vi "vision map lines.vi"(10 "GIC Input":T2={"     Use ?\nOff       On"=[FALSE, TRUE, FALSE, TRUE], "Mode:"=FALSE, "Extra Port"="", "Hokuyo Port"="COM7", "Tx Prop  Port"="COM6", "Compass Port"="", "GPS Port"="", "Num of WPs"=0, "WP Lats and Longs"={"WP Lats"=[], "WP Longs"=[]}, "Obst Lats and Longs"={"Obst Lats"=[], "Obst Longs"=[]}, "Parameters"=[], "GPS Data"=[], "Compass"=0.0, "LMS Vector"=[], "Vision Vector"=[], "Direction Cmd"=0.0, "Speed Cmd"=0.0, "WP Vector"=[], "WP Number"=0, "Extra"=0, "SW Map"=[], "Path Cluster"={"Path x node"=[], "Path y node"=[]}, "Sim Course"=[]} {"Obst Lats and Longs"."Obst Longs" format="%#_8g"; "Obst Lats and Longs"."Obst Lats" format="%#_8g"}) -> (2 "GIC Output":T1={"     Use ?\nOff       On"=[FALSE, TRUE, FALSE, TRUE], "Mode:"=FALSE, "Extra Port"="", "Hokuyo Port"="COM7", "Tx Prop Port"="COM6", "Compass Port"="", "GPS Port"="", "Num of WPs"=0, "WP Lats and Longs"={"WP Lats"=[], "WP Longs"=[]}, "Obst Lats and Longs"={"Obst Lats"=[], "Obst Longs"=[]}, "Parameters"=[], "GPS Data"=[], "Compass"=0.0, "LMS Vector"=[], "Vision Vector"=[], "Direction Cmd"=0.0, "Speed Cmd"=0.0, "WP Vector"=[], "WP Number"=0, "Extra"=0, "SW Map"=[], "Path Cluster"={"Path x node"=[], "Path y node"=[]}, "Sim Course"=[]} {"Obst Lats and Longs"."Obst Longs" format="%#_8g"; "Obst Lats and Longs"."Obst Lats" format="%#_8g"})   [LabVIEW 2014]
panel:
  in  "y4":dbl
  in  "x4":dbl
  in  "y3":dbl
  in  "x3":dbl
  in  "y2":dbl
  in  "x2":dbl
  in  "y1":dbl
  in  "x1":dbl
  out "Local Map":picture
  out "slope":dbl
  out "yn4":dbl
  out "xn4":dbl
  out "yn3":dbl
  out "xn3":dbl
  out "yn2":dbl
  out "xn2":dbl
  out "yn1":dbl
  out "xn1":dbl
  out "th":dbl
  out "ppm":dbl
  out "yp":dbl
  out "xp":dbl
  out "SwMap out":dbl[][](array[numeric])
  # "Vision Map Lines"
  # "Input:"
  # "Output"
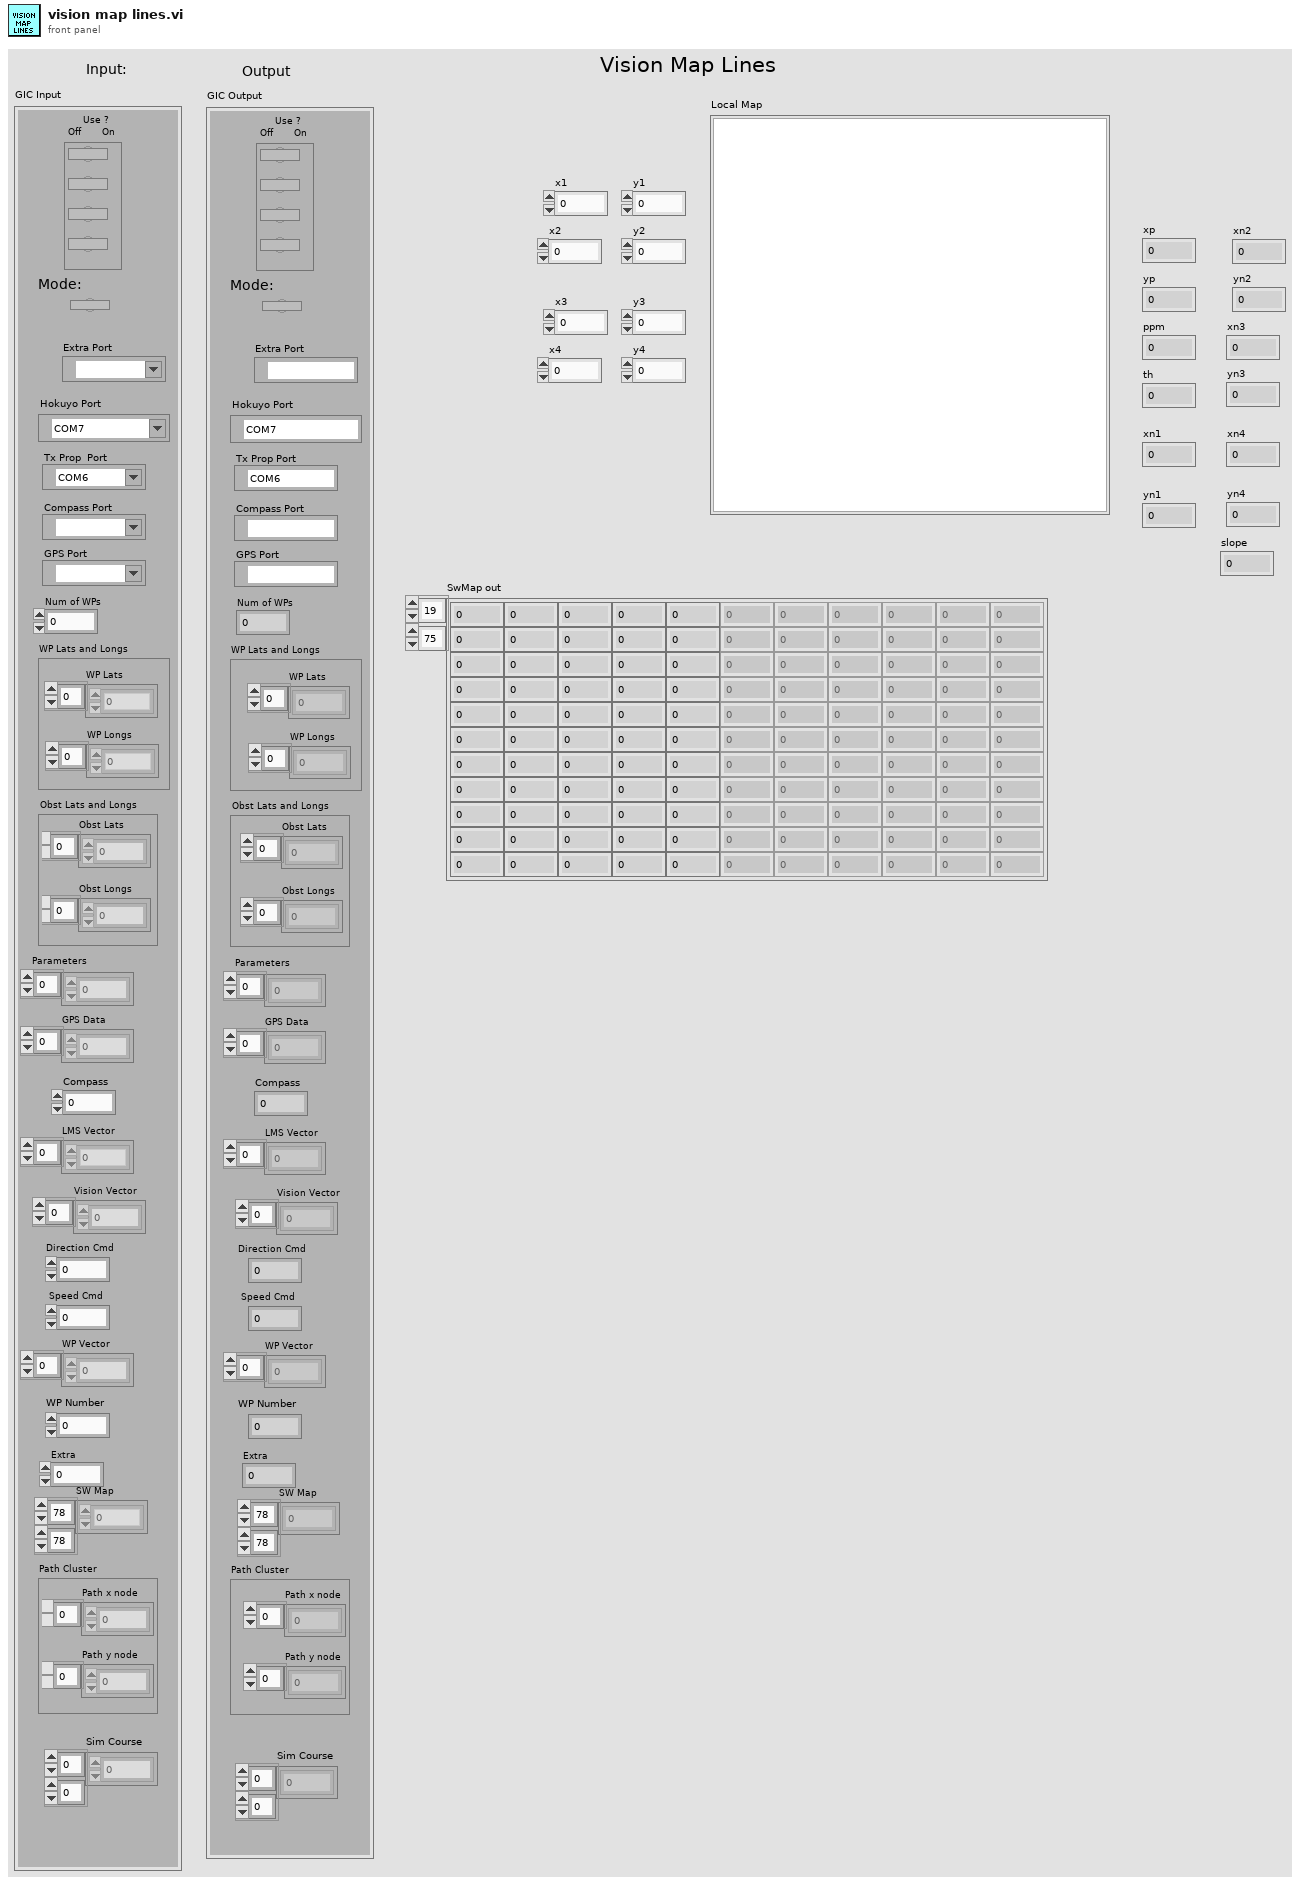
[diagram p1: front panel]
types:
  T1 = cluster{"     Use ?\nOff       On":bool[], "Mode:":bool, "Extra Port":refnum<visa-resource-name>, "Hokuyo Port":refnum<visa-resource-name>, "Tx Prop Port":refnum<visa-resource-name>, "Compass Port":refnum<visa-resource-name>, "GPS Port":refnum<visa-resource-name>, "Num of WPs":i16, "WP Lats and Longs":cluster{"WP Lats":dbl[], "WP Longs":dbl[]}, "Obst Lats and Longs":cluster{"Obst Lats":dbl[], "Obst Longs":dbl[]}, "Parameters":dbl[], "GPS Data":dbl[], "Compass":dbl, "LMS Vector":dbl[], "Vision Vector":dbl[], "Direction Cmd":dbl, "Speed Cmd":dbl, "WP Vector":dbl[], "WP Number":i32, "Extra":i16, "SW Map":i32[][], "Path Cluster":cluster{"Path x node":dbl[], "Path y node":dbl[]}, "Sim Course":i8[][]}
  T2 = cluster{"     Use ?\nOff       On":bool[], "Mode:":bool, "Extra Port":refnum<visa-resource-name>, "Hokuyo Port":refnum<visa-resource-name>, "Tx Prop  Port":refnum<visa-resource-name>, "Compass Port":refnum<visa-resource-name>, "GPS Port":refnum<visa-resource-name>, "Num of WPs":i16, "WP Lats and Longs":cluster{"WP Lats":dbl[], "WP Longs":dbl[]}, "Obst Lats and Longs":cluster{"Obst Lats":dbl[], "Obst Longs":dbl[]}, "Parameters":dbl[], "GPS Data":dbl[], "Compass":dbl, "LMS Vector":dbl[], "Vision Vector":dbl[], "Direction Cmd":dbl, "Speed Cmd":dbl, "WP Vector":dbl[], "WP Number":i32, "Extra":i16, "SW Map":i32[][], "Path Cluster":cluster{"Path x node":dbl[], "Path y node":dbl[]}, "Sim Course":i8[][]}
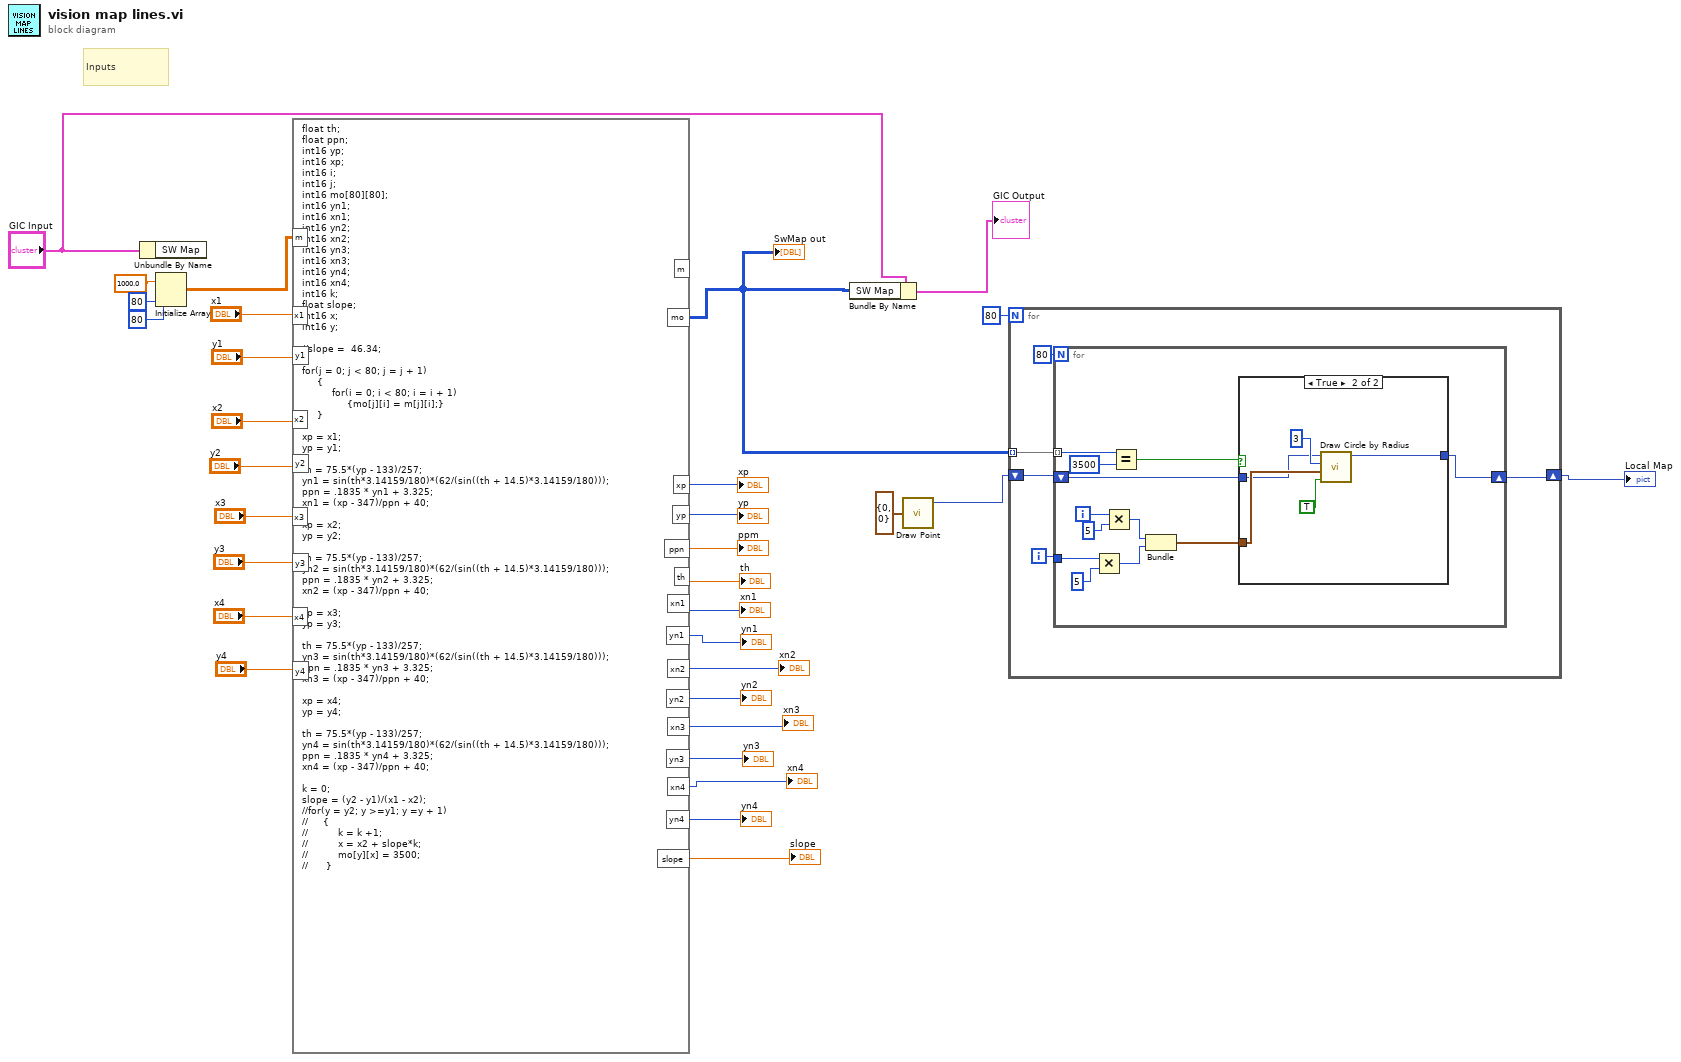
[diagram p0: block diagram]
diagram:
  # "Inputs"
  n1 = Unbundle By Name("GIC Input") -> ()  [unwired: 1 out]
  n2 = Initialize Array(1000.0 ("element"), 80 ("dimension size"), 80 ("dimension size")) -> (w1:dbl[][])
  n3 = formula code="float th;   \nfloat ppn;  \nint16 yp;\nint16 xp;\nint16 i;\nint16 j;\nint16 mo[80][80];\nint16 yn1;\nint16 xn1;\nint16 yn2;\nint16 xn2;\nint16 yn3;\nint16 xn3;\nint16 yn4;\nint16 xn4;\nint16 k;\nfloat slope;\nint16 x;\nint16 y;\n\n//slope =  46.34;\n\nfor(j = 0; j < 80; j = j + 1)\n     {\n          for(i = 0; i < 80; i = i + 1)\n               {mo[j][i] = m[j][i];}\n     }\n\nxp = x1;\nyp = y1;\n\nth = 75.5*(yp - 133)/257;\nyn1 = sin(th*3.14159/180)*(62/(sin((th + 14.5)*3.14159/180)));\nppn = .1835 * yn1 + 3.325;\nxn1 = (xp - 347)/ppn + 40;\n\nxp = x2;\nyp = y2;\n\nth = 75.5*(yp - 133)/257;\nyn2 = sin(th*3.14159/180)*(62/(sin((th + 14.5)*3.14159/180)));\nppn = .1835 * yn2 + 3.325;\nxn2 = (xp - 347)/ppn + 40;\n\nxp = x3;\nyp = y3;\n\nth = 75.5*(yp - 133)/257;\nyn3 = sin(th*3.14159/180)*(62/(sin((th + 14.5)*3.14159/180)));\nppn = .1835 * yn3 + 3.325;\nxn3 = (xp - 347)/ppn + 40;\n\nxp = x4;\nyp = y4;\n\nth = 75.5*(yp - 133)/257;\nyn4 = sin(th*3.14159/180)*(62/(sin((th + 14.5)*3.14159/180)));\nppn = .1835 * yn4 + 3.325;\nxn4 = (xp - 347)/ppn + 40;\n\nk = 0;\nslope = (y2 - y1)/(x1 - x2);\n//for(y = y2; y >=y1; y =y + 1)\n//     {\n//          k = k +1;\n//          x = x2 + slope*k;\n//          mo[y][x] = 3500;\n//      }"("m"=w1, "x1"="x1", "y1"="y1", "x2"="x2", "y2"="y2", "x3"="x3", "y3"="y3", "x4"="x4", "y4"="y4") -> ("mo"=w11:i16[][], "xp"=→"xp":i16, "yp"=→"yp":i16, "ppn"=→"ppm":dbl, "th"=→"th":dbl, "xn1"=→"xn1":i16, "yn1"=→"yn1":i16, "xn2"=→"xn2":i16, "yn2"=→"yn2":i16, "xn3"=→"xn3":i16, "yn3"=→"yn3":i16, "xn4"=→"xn4":i16, "yn4"=→"yn4":i16, "slope"=→"slope":dbl)  [unwired: 1 out]
  "SwMap out" <- w11
  n4 = Bundle By Name(cluster="GIC Input", "SW Map"=w11) -> (→"GIC Output":T2)
  n5 = call <vilib>:"Draw Point.vi"("point(x,y)"=cluster{"x":i16, "y":i16} {"x"=0, "y"=0}) -> ("new picture"=w14:picture)  [unwired: 8 in]
  n6 = for {
    N: 80 -> [_]
    tunnel: w11 -> [w36] mode=indexing
    shift-right: [w34] -> w15
    shift-left: w14 -> [w33]
    i -> [w35]
    n7 = for {
      N: 80 -> [_]
      tunnel: w36 -> [w49] mode=indexing
      tunnel: w35 -> [w44]
      shift-right: [w39] -> w34
      shift-left: w33 -> [w38]
      i -> [w46]
      n8 = Multiply(x=w44, y=5) -> (x*y=w41:i32)
      n9 = Multiply(x=w46, y=5) -> (x*y=w42:i32)
      n10 = Equal?(x=w49, y=i16 3500) -> (x = y?=w47:bool)
      n11 = Bundle(w42, w41) -> (w40:cluster{i32, i32})  [unwired: 1 in]
      n12 = case shown="True" w47 {
        tunnel: w40 -> [_ w53]
        tunnel: [w50 w52] -> w39
        tunnel: w38 -> [w50 w51]
        frame False {
        }
        frame True {
          n13 = call <vilib>:"Draw Circle by Radius.vi"("fill?(F)"=TRUE, "pixel center"=w53, "radius"=i16 3, "picture"=w51) -> ("new picture"=w52:picture)  [unwired: 7 in]
        }
      }
    }
  }
  "Local Map" <- w15
